vi "QDMH POLY Enqueue String.vi"(8 "error in (no error)":errorcluster, 10 "State":string, 11 "queue":refnum<queue>) -> (0 "error out":errorcluster, 3 "queue out":refnum<queue>)   [LabVIEW 2019]
doc: "This is an instance VI for the polymorphic enqueue VI.\n\nAAL 9/09"
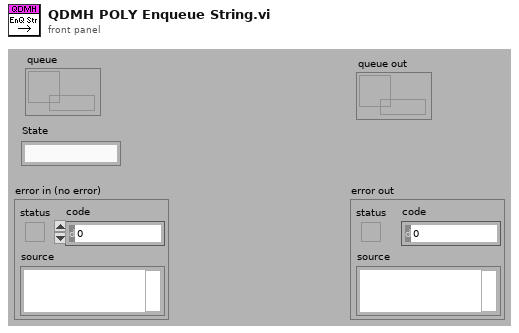
[diagram p1: front panel]
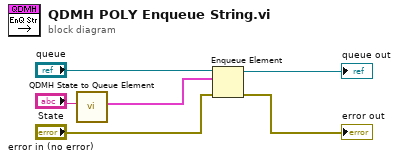
[diagram p0: block diagram]
diagram:
  n1 = call "QDMH State to Queue Element.vi"("State"="State") -> ("QDSM Element"=w4:cluster{"State":string, "Variant Data":variant})  [unwired: 10 out]
  n2 = Enqueue Element(queue="queue", element=w4, error in (no error)="error in (no error)") -> (queue out=→"queue out":refnum<queue>, error out=→"error out":errorcluster)  [unwired: 2 out]
